vi "write.vi"(8 "error in (no error)":errorcluster, 10 "Data":u8[](array[numeric]), 11 "M1M3SAL in":refnum<class "M1M3SAL.lvclass">) -> (0 "error out":errorcluster, 3 "M1M3SAL out":refnum<class "M1M3SAL.lvclass">)   [LabVIEW 2016, in "M1M3SAL.lvlib" / "M1M3SAL.lvclass"]
uses:
  M1M3SAL.lvclass
  M1M3SAL.lvclass/M1M3SAL.ctl
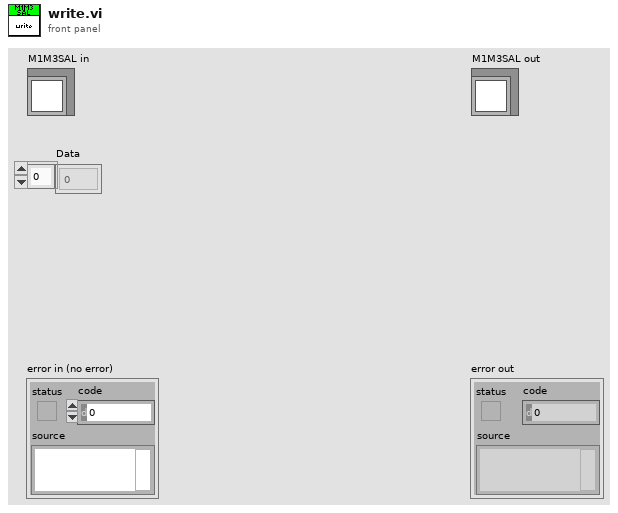
[diagram p1: front panel]
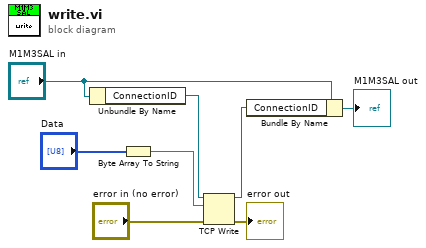
[diagram p0: block diagram]
diagram:
  n1 = Unbundle By Name("M1M3SAL in") -> ("ConnectionID"=w6:refnum<k5>)
  n2 = Byte Array To String(unsigned byte array="Data") -> (string=w3:string)
  n3 = TCP Write(connection ID=w6, data in=w3, error in (no error)="error in (no error)") -> (connection ID out=w5:refnum<k5>, error out=→"error out":errorcluster)  [unwired: 1 in, 1 out]
  n4 = Bundle By Name(cluster="M1M3SAL in", "ConnectionID"=w5) -> (→"M1M3SAL out":refnum<class "M1M3SAL.lvclass">)
